vi "Create new array.vi"(8 "Numeric":i32, 10 "Array 2":cluster{dbl[], dbl[]}[](array[cluster]), 11 "A vs D":cluster{dbl[], dbl[]}[](array[cluster])) -> (3 "Array":cluster{dbl[], dbl[]}[](array[cluster]))   [LabVIEW 2016]
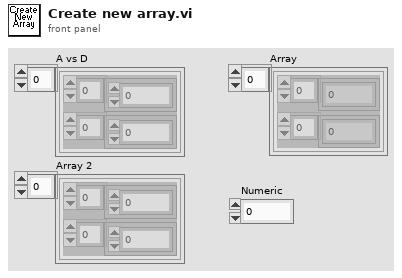
[diagram p1: front panel]
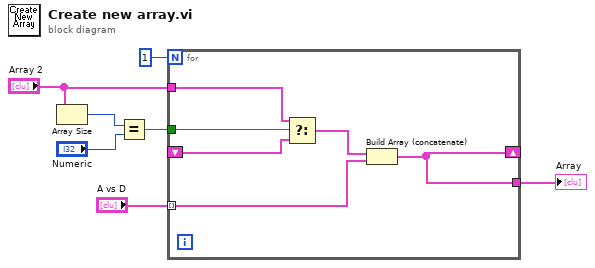
[diagram p0: block diagram]
diagram:
  n1 = Array Size(array="Array 2") -> (size(s)=w4:i32)
  n2 = Equal?(x=w4, y="Numeric") -> (x = y?=w1:bool)
  n3 = for {
    N: 1 -> [_]
    tunnel: "A vs D" -> [w13] mode=indexing
    shift-right: [w12] -> _
    shift-left: _ -> [w10]
    tunnel: [w12] -> w7
    tunnel: "Array 2" -> [w11]
    tunnel: w1 -> [w9]
    n4 = Select(t=w11, s=w9, f=w10) -> (s? t:f=w8:cluster{dbl[], dbl[]}[])
    n5 = Build Array (concatenate)(w8, w13) -> (w12:cluster{dbl[], dbl[]}[])
  }
  "Array" <- w7
